vi "Wait on listenner.vi"(8 "error in (no error)":errorcluster, 11 "Server in":refnum<class "TCP-Server.lvclass">) -> (0 "error out":errorcluster, 3 "Server out":refnum<class "TCP-Server.lvclass">)   [LabVIEW 2018, in "TCP-Server.lvclass"]
uses:
  TCP-Server.lvclass
  TCP-Server.lvclass/TCP-Server.ctl
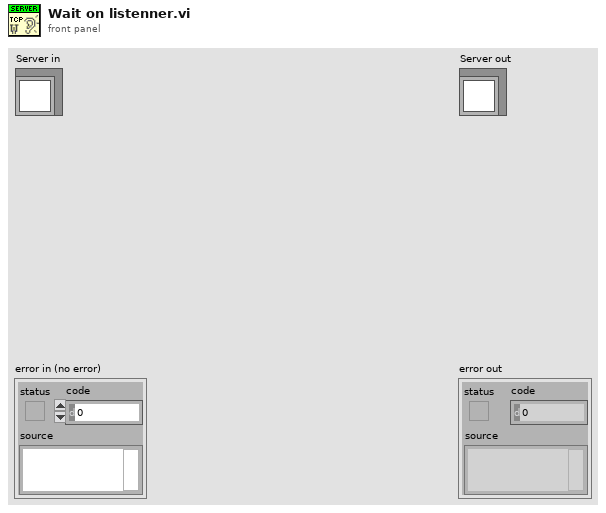
[diagram p1: front panel]
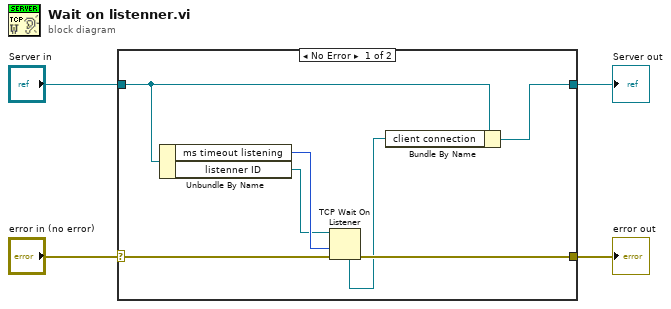
[diagram p0: block diagram]
diagram:
  n1 = case shown="No Error" "error in (no error)" {
    selector: "error in (no error)" -> [w11 w12]
    tunnel: [w8 w12] -> w3
    tunnel: [w6 w13] -> w1
    tunnel: "Server in" -> [w7 w13]
    frame No Error {
      n2 = Unbundle By Name(w7) -> ("ms timeout listening"=w10:i32, "listenner ID"=w9:refnum<k5>)
      n3 = TCP Wait On Listener(8:w11, 9:w10, 11:w9) -> (0:w8:errorcluster, 4:w5:refnum<k5>)  [unwired: 1 in, 3 out]
      n4 = Bundle By Name(cluster=w7, "client connection"=w5) -> (w6:refnum<class "TCP-Server.lvclass">)
    }
    frame Error {
    }
  }
  "error out" <- w3
  "Server out" <- w1
